vi "Log Errors.vi"(1 "Error Queue":refnum<queue>, 2 "Error Notifier":refnum<notifier>, 3 "Log File Cluster":T1) -> ()   [LabVIEW 2016]
uses:
  Log File Cluster.ctl
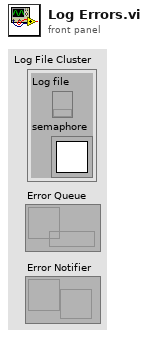
[diagram p1: front panel]
types:
  T1 = typedef "Log File Cluster.ctl" = cluster{"Log file":refnum<k34>, "semaphore":T2}
  T2 = typedef "Semaphore RefNum" = refnum<k1>
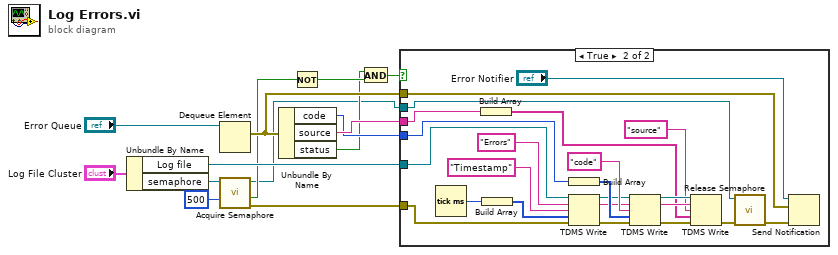
[diagram p0: block diagram]
diagram:
  n1 = Unbundle By Name("Log File Cluster") -> ("Log file"=w12:refnum<k34>, "semaphore"=w8:T2)
  n2 = Dequeue Element(queue="Error Queue") -> (element=w11:errorcluster)  [unwired: 2 in, 3 out]
  n3 = call <vilib>:"Acquire Semaphore.vi"("ms timeout (-1)"=500, "semaphore"=w8) -> ("error out"=w3:errorcluster, "timed out"=w7:bool, "semaphore out"=w2:T2)  [unwired: 3 in]
  n4 = Unbundle By Name(w11) -> ("code"=w9:i32, "source"=w10:string, "status"=w5:bool)
  n5 = Not(x=w7) -> (.not. x?=w6:bool)
  n6 = And(x=w5, y=w6) -> (x .and. y?=w4:bool)
  n7 = case shown="True" w4 {
    tunnel: w12 -> [_ w23]
    tunnel: w11 -> [_ w21]
    tunnel: w10 -> [_ w19]
    tunnel: w9 -> [_ w18]
    tunnel: w3 -> [_ w16]
    tunnel: w2 -> [_ w15]
    frame False {
    }
    frame True {
      n8 = Tick Count (ms)() -> (millisecond timer value=w30:u32)
      n9 = Build Array(w19) -> (w33:string[])
      n10 = Build Array(w30) -> (w29:u32[])
      n11 = Build Array(w18) -> (w37:i32[])
      n12 = TDMS Write(0:w23, 5:"Errors" ("group name in (Untitled)"), 7:"Timestamp", 9:w29, 11:w16) -> (4:w24:refnum<k34>, 6:w26:string, 15:w25:errorcluster)  [unwired: 1 in, 1 out]
      n13 = TDMS Write(0:w24, 5:w26, 7:"code", 9:w37, 11:w25) -> (4:w36:refnum<k34>, 6:w35:string, 15:w34:errorcluster)  [unwired: 1 in, 1 out]
      n14 = TDMS Write(0:w36, 5:w35, 7:"source", 9:w33, 11:w34) -> (15:w22:errorcluster)  [unwired: 1 in, 3 out]
      n15 = call <vilib>:"Release Semaphore.vi"("error in (no error)"=w22, "semaphore"=w15) -> ("error out"=w17:errorcluster)  [unwired: 4 in, 1 out]
      n16 = Send Notification(notification=w21, notifier="Error Notifier", error in (no error)=w17) -> ()  [unwired: 2 out]
    }
  }
